vi "Prasing Frame.vi"(8 "error in (no error)":errorcluster caption="entrée d'erreur (pas d'erreur)", 11 "Class UART Enocean en entrée":refnum<class "Class UART P2056.lvclass">) -> (0 "error out":errorcluster caption="sortie d'erreur", 3 "Class UART Enocean en sortie":refnum<class "Class UART P2056.lvclass">)   [LabVIEW 2020, in "Library Instrument & Equipement.lvlib" / "Library UART.lvlib" / "Class UART P2056.lvclass"]
uses:
  Class UART P2056.lvclass
  C:/Users/ngarcin/OneDrive - Altyor/Standard TB/Class/UART/UART (Default)/Class UART (Default).lvclass
  Class UART P2056.lvclass/Class UART P2056.ctl
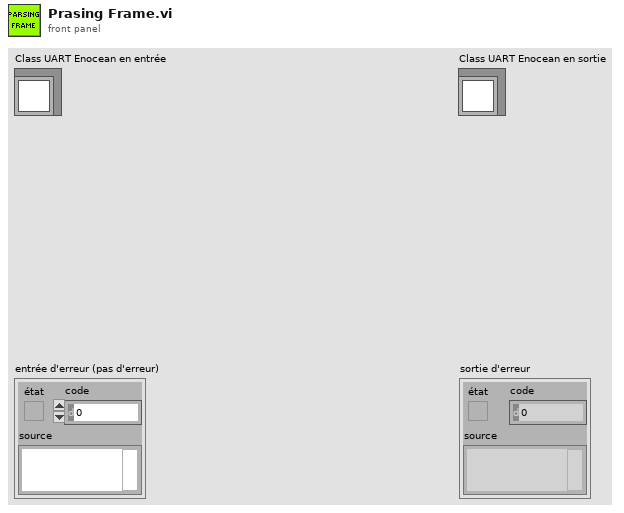
[diagram p1: front panel]
types:
  T1 = enum16{"Wait Data Start", "Wait Lenght", "Read Data", "Wait Size Data"}[]
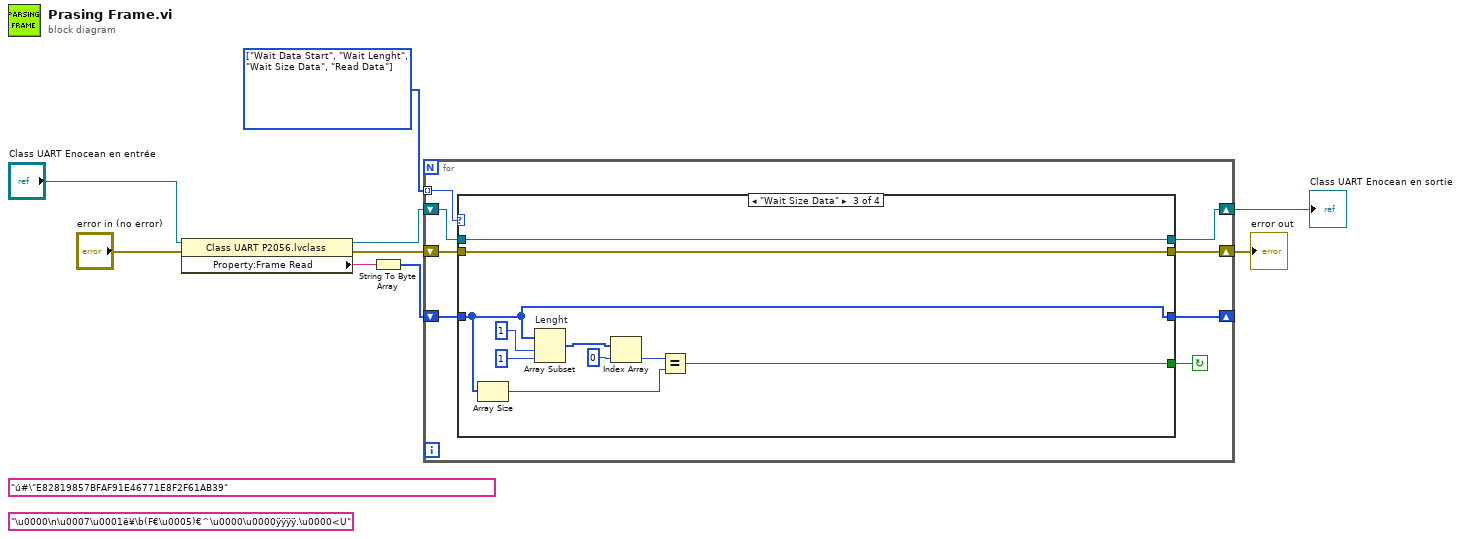
[diagram p0: block diagram]
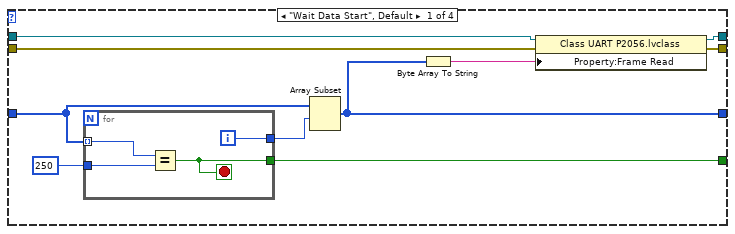
[diagram p2: hidden frame]
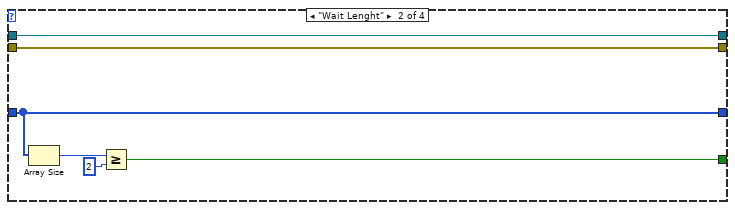
[diagram p3: hidden frame]
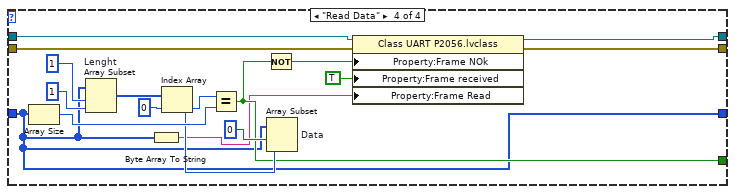
[diagram p4: hidden frame]
diagram:
  (unwired) "\u0000\n\u0007\u0001ë¥\b(F€\u0005)€^\u0000\u0000ÿÿÿÿ.\u0000<U" ("chaîne")
  (unwired) "ú#\"E82819857BFAF91E46771E8F2F61AB39" ("chaîne")
  w7 = T1 [enum."Wait Data Start", enum."Wait Lenght", enum."Wait Size Data", enum."Read Data"] items=["Wait Data Start", "Wait Lenght", "Read Data", "Wait Size Data"]
  n1 = property class="Class UART P2056.lvclass"(reference="Class UART Enocean en entrée", error in="error in (no error)") -> (reference out=w5:refnum<class "Class UART P2056.lvclass">, error out=w2:errorcluster, "Property:Frame Read"=w1:string)
  n2 = String To Byte Array(string=w1) -> (unsigned byte array=w6:u8[])
  n3 = for {
    tunnel: w7 -> [w16] mode=indexing
    shift-right: [w13] -> w4
    shift-left: w5 -> [w14]
    shift-right: [w11] -> w3
    shift-left: w2 -> [w12]
    shift-right: [w10] -> _
    shift-left: w6 -> [w17]
    stop <- w15 continue-if-true
    n4 = case shown="\"Wait Size Data\"" w16 {
      tunnel: w17 -> [w21 w37 w42 w50]
      tunnel: [w26 w34 w38 w52] -> w15
      tunnel: w14 -> [w25 w33 w47 w61]
      tunnel: [w24 w33 w47 w58] -> w13
      tunnel: w12 -> [w23 w32 w46 w60]
      tunnel: [w22 w32 w46 w59] -> w11
      tunnel: [w18 w37 w42 w50] -> w10
      frame "Wait Data Start", Default {
        n5 = for {
          tunnel: w21 -> [w31] mode=indexing
          tunnel: [w30] -> w20
          tunnel: u8 250 -> [w29]
          tunnel: [w28] -> w26
          i -> [w30]
          stop <- w28 stop-if-true
          n6 = Equal?(x=w31, y=w29) -> (x = y?=w28:bool)
        }
        n7 = Array Subset(array=w21, index=w20) -> (w18:u8[])  [unwired: 1 in]
        n8 = Byte Array To String(unsigned byte array=w18) -> (string=w19:string)
        n9 = property class="Class UART P2056.lvclass"(reference=w25, error in=w23, "Property:Frame Read"=w19) -> (reference out=w24:refnum<class "Class UART P2056.lvclass">, error out=w22:errorcluster)
      }
      frame "Wait Lenght" {
        n10 = Array Size(array=w37) -> (size(s)=w36:i32)
        n11 = Greater Or Equal?(x=w36, y=2) -> (x >= y?=w34:bool)
      }
      frame "Wait Size Data" {
        n12 = Array Size(array=w42) -> (size(s)=w41:i32)
        n13 = Array Subset "Lenght"(array=w42, index=1 ("indice"), length=1 ("longueur")) -> (w43:u8[])
        n14 = Index Array(array=w43, index=0 ("indice")) -> (element=w40:u8)
        n15 = Equal?(x=w40, y=w41) -> (x = y?=w38:bool)
      }
      frame "Read Data" {
        n16 = Array Size(array=w50) -> (size(s)=w54:i32)
        n17 = Array Subset "Lenght"(array=w50, index=1 ("indice"), length=1 ("longueur")) -> (w57:u8[])
        n18 = Byte Array To String(unsigned byte array=w50) -> (string=w51:string)
        n19 = Index Array(array=w57, index=0 ("indice")) -> (element=w53:u8)
        n20 = Equal?(x=w53, y=w54) -> (x = y?=w52:bool)
        n21 = Not(x=w52) -> (.not. x?=w49:bool)
        n22 = Array Subset "Data"(array=w50, index=0 ("indice"), length=w53) -> ()  [unwired: 1 out]
        n23 = property class="Class UART P2056.lvclass"(reference=w61, error in=w60, "Property:Frame NOk"=w49, "Property:Frame received"=TRUE ("Frame received"), "Property:Frame Read"=w51) -> (reference out=w58:refnum<class "Class UART P2056.lvclass">, error out=w59:errorcluster)
      }
    }
  }
  "error out" <- w3
  "Class UART Enocean en sortie" <- w4
